vi "Load_TimeTable.vi"(7 "ReadOnly":T11={"Qref"={"ValveCTR"=refnum, "Error"=refnum}, "UI_EN"=FALSE, "UserEventREF"={"TimeBasedProducer"={"Reg"=refnum, "Ref"=refnum}, "TimeBasedTempRead"={"Reg"=refnum, "Ref"=refnum}}, "UI_REF"=variant, "Paths"={"Log_Dir"=path "", "TempLog"=path "", "WateringLog"=path "", "Error"=path "", "Settings_Dir"=path "", "CFG.ini"=path "", "Plant_Digital_OP"=path "", "TimeTable"=path "", "Consol_Dir"=path "", "Input"=path "", "Output"=path "", "Timeout"=path "", "TimeoutTable"=path "", "Ch_Stat"=path "", "Temp"=path ""}, "PI_REF"={"IO"=enum."Remote", "Interface"=enum."Serial", "LINX Device Config"={"Interface"=enum."Serial", "COM Port"="COM13", "TCP Configuration"={"IP Address"="", "Port"=0}, "Device Family"=1, "Device ID"=1, "Device Name"="myRIO-1900", "TCP Ref"=refnum, "Channels"={"DI"=[0, 1, 2, 3, 4, 5, 6, 7, 8, 9, 10, 11, 12, 13, 14, 15, 16, 17, 18, 19, 20, 21, 22, 23, 24, 25, 26, 27, 28, 29, 30, 31, 32, 33, 34, 35, 36, 37, 38, 39, 40, 41, 42, 43, 44, 45, 46], "DO"=[0, 1, 2, 3, 4, 5, 6, 7, 8, 9, 10, 11, 12, 13, 14, 15, 16, 17, 18, 19, 20, 21, 22, 23, 24, 25, 26, 27, 28, 29, 30, 31, 32, 33, 34, 35, 36, 37, 38, 39, 40, 41, 42, 43, 44, 45, 46], "AI"=[0, 1, 2, 3, 4, 5, 6, 7, 8, 9, 10, 11], "AO"=[], "PWM"=[3, 5, 6, 9, 10], "QE"=[], "UART"=[0, 1], "I2C 2"=[0], "SPI"=[0], "CAN"=[], "Servo"=[], "AI Ref (V)"=0.0, "AI Resolution (Bits)"=0, "AO Ref (V)"=0.0, "AO Resolution (Bits)"=0}}}, "CFG"={"ProducerEn_PC"=FALSE, "Producer_PC_ms"=0, "ProducerEn_PI"=FALSE, "Producer_PI_ms"=0, "TempLogInterval"=15, "SystemResetTime"=0.0}} {"CFG"."SystemResetTime" format="%<%H:%M:%S>t"}, 8 "Error In":errorcluster, 10 "Time Table":refnum<vi>, 11 "Read_WriteIN":T1={"Time Table"=[{"Set Time"=0.0, "Control"=enum."Time", "Duration[S]"=3.0, "Liter"=0.0, "Plant Name."="", "Watered"=FALSE, "Su"=FALSE, "Mo"=FALSE, "Tu"=FALSE, "We"=FALSE, "Th"=FALSE, "Fr"=FALSE, "Sa"=FALSE}, {"Set Time"=0.0, "Control"=enum."Time", "Duration[S]"=5.0, "Liter"=0.0, "Plant Name."="", "Watered"=FALSE, "Su"=FALSE, "Mo"=FALSE, "Tu"=FALSE, "We"=FALSE, "Th"=FALSE, "Fr"=FALSE, "Sa"=FALSE}, {"Set Time"=0.0, "Control"=enum."Time", "Duration[S]"=5.0, "Liter"=0.0, "Plant Name."="", "Watered"=FALSE, "Su"=FALSE, "Mo"=FALSE, "Tu"=FALSE, "We"=FALSE, "Th"=FALSE, "Fr"=FALSE, "Sa"=FALSE}], "Plants_Digital_OP"=[], "delta_ms_w_Index"={"delta_ms"=[], "Index"=[], "RunArray"=[]}, "TimeOutInfo"={"Timeout"=0, "ValveCTR"={"State"=enum."Open Valve", "Channel No"=0, "Duration[S]"=0.0}, "Index"=0}, "LoopName"=""} {"TimeOutInfo"."ValveCTR"."Channel No" items=["7"=7, "11"=11, "12"=12, "13"=13, "15"=15, "16"=16, "18"=18, "29"=29, "32"=32, "33"=33, "35"=35, "36"=36, "37"=37, "38"=38, "40"=40]; "delta_ms_w_Index"."RunArray"."Channel No" items=["7"=7, "11"=11, "12"=12, "13"=13, "15"=15, "16"=16, "18"=18, "29"=29, "32"=32, "33"=33, "35"=35, "36"=36, "37"=37, "38"=38, "40"=40]; "Plants_Digital_OP"."Channel No" items=["7"=7, "11"=11, "12"=12, "13"=13, "15"=15, "16"=16, "18"=18, "29"=29, "32"=32, "33"=33, "35"=35, "36"=36, "37"=37, "38"=38, "40"=40]; "Time Table"."Liter" min=0.0; "Time Table"."Set Time" format="%<%H:%M:%S>t"; "Time Table"."Duration[S]" min=0.0}) -> (0 "Error Out":errorcluster, 3 "Read_WriteIOUT":T1={"Time Table"=[{"Set Time"=0.0, "Control"=enum."Time", "Duration[S]"=3.0, "Liter"=0.0, "Plant Name."="", "Watered"=FALSE, "Su"=FALSE, "Mo"=FALSE, "Tu"=FALSE, "We"=FALSE, "Th"=FALSE, "Fr"=FALSE, "Sa"=FALSE}, {"Set Time"=0.0, "Control"=enum."Time", "Duration[S]"=5.0, "Liter"=0.0, "Plant Name."="", "Watered"=FALSE, "Su"=FALSE, "Mo"=FALSE, "Tu"=FALSE, "We"=FALSE, "Th"=FALSE, "Fr"=FALSE, "Sa"=FALSE}, {"Set Time"=0.0, "Control"=enum."Time", "Duration[S]"=5.0, "Liter"=0.0, "Plant Name."="", "Watered"=FALSE, "Su"=FALSE, "Mo"=FALSE, "Tu"=FALSE, "We"=FALSE, "Th"=FALSE, "Fr"=FALSE, "Sa"=FALSE}], "Plants_Digital_OP"=[], "delta_ms_w_Index"={"delta_ms"=[], "Index"=[], "RunArray"=[]}, "TimeOutInfo"={"Timeout"=0, "ValveCTR"={"State"=enum."Open Valve", "Channel No"=0, "Duration[S]"=0.0}, "Index"=0}, "LoopName"=""} {"TimeOutInfo"."ValveCTR"."Channel No" items=["7"=7, "11"=11, "12"=12, "13"=13, "15"=15, "16"=16, "18"=18, "29"=29, "32"=32, "33"=33, "35"=35, "36"=36, "37"=37, "38"=38, "40"=40]; "delta_ms_w_Index"."RunArray"."Channel No" items=["7"=7, "11"=11, "12"=12, "13"=13, "15"=15, "16"=16, "18"=18, "29"=29, "32"=32, "33"=33, "35"=35, "36"=36, "37"=37, "38"=38, "40"=40]; "Plants_Digital_OP"."Channel No" items=["7"=7, "11"=11, "12"=12, "13"=13, "15"=15, "16"=16, "18"=18, "29"=29, "32"=32, "33"=33, "35"=35, "36"=36, "37"=37, "38"=38, "40"=40]; "Time Table"."Liter" min=0.0; "Time Table"."Set Time" format="%<%H:%M:%S>t"; "Time Table"."Duration[S]" min=0.0})   [LabVIEW 2014, in "TimeBasedProd.lvlib"]
uses:
  TimeBasedProd.lvlib
  Main/TypeDef/ReadOnly.ctl
  ValveCTRL/TypeDef/Queue_Cluster.ctl
  ValveCTRL/TypeDef/States_Enum.ctl
  ValveCTRL/TypeDef/CHs_List.ctl
  Main/TypeDef/EventData.ctl
  <vilib>/MakerHub/LINX/Private/Type Defs/LINX Ref.ctl
  <vilib>/MakerHub/LINX/Private/Type Defs/Platform.ctl
  <vilib>/MakerHub/LINX/Private/Type Defs/Interface.ctl
  <vilib>/MakerHub/LINX/Private/Device/Type Defs/LINX Device Config.ctl
  <vilib>/MakerHub/LINX/Private/Device/Type Defs/TCP Config.ctl
  <vilib>/MakerHub/LINX/Private/Device/Type Defs/Channels.ctl
  Main/Init/ReadInitCFG/TypeDef/CFG_Cluster.ctl
  TypeDef/Read_Write.ctl
  TypeDef/Time_Table.ctl
  TypeDef/Time_Table_CTR.ctl
  Digital_OP/TypeDef/Plant_OP_Map.ctl
  Digital_OP/TypeDef/Plant_OP_Map_CTR.ctl
  TypeDef/TimeOutInfo.ctl
  TypeDef/UpdateTimeOutinfo.ctl
  ValveCTRL/ValveCTRL.lvlib
  Main/Main.lvlib
  <vilib>/MakerHub/LINX/LMH-LINX.lvlib
  <vilib>/MakerHub/LINX/Private/Device/Device.lvlib
panel:
  # "Watering Days"
  # "Watering Days"
  # "Watering Days"
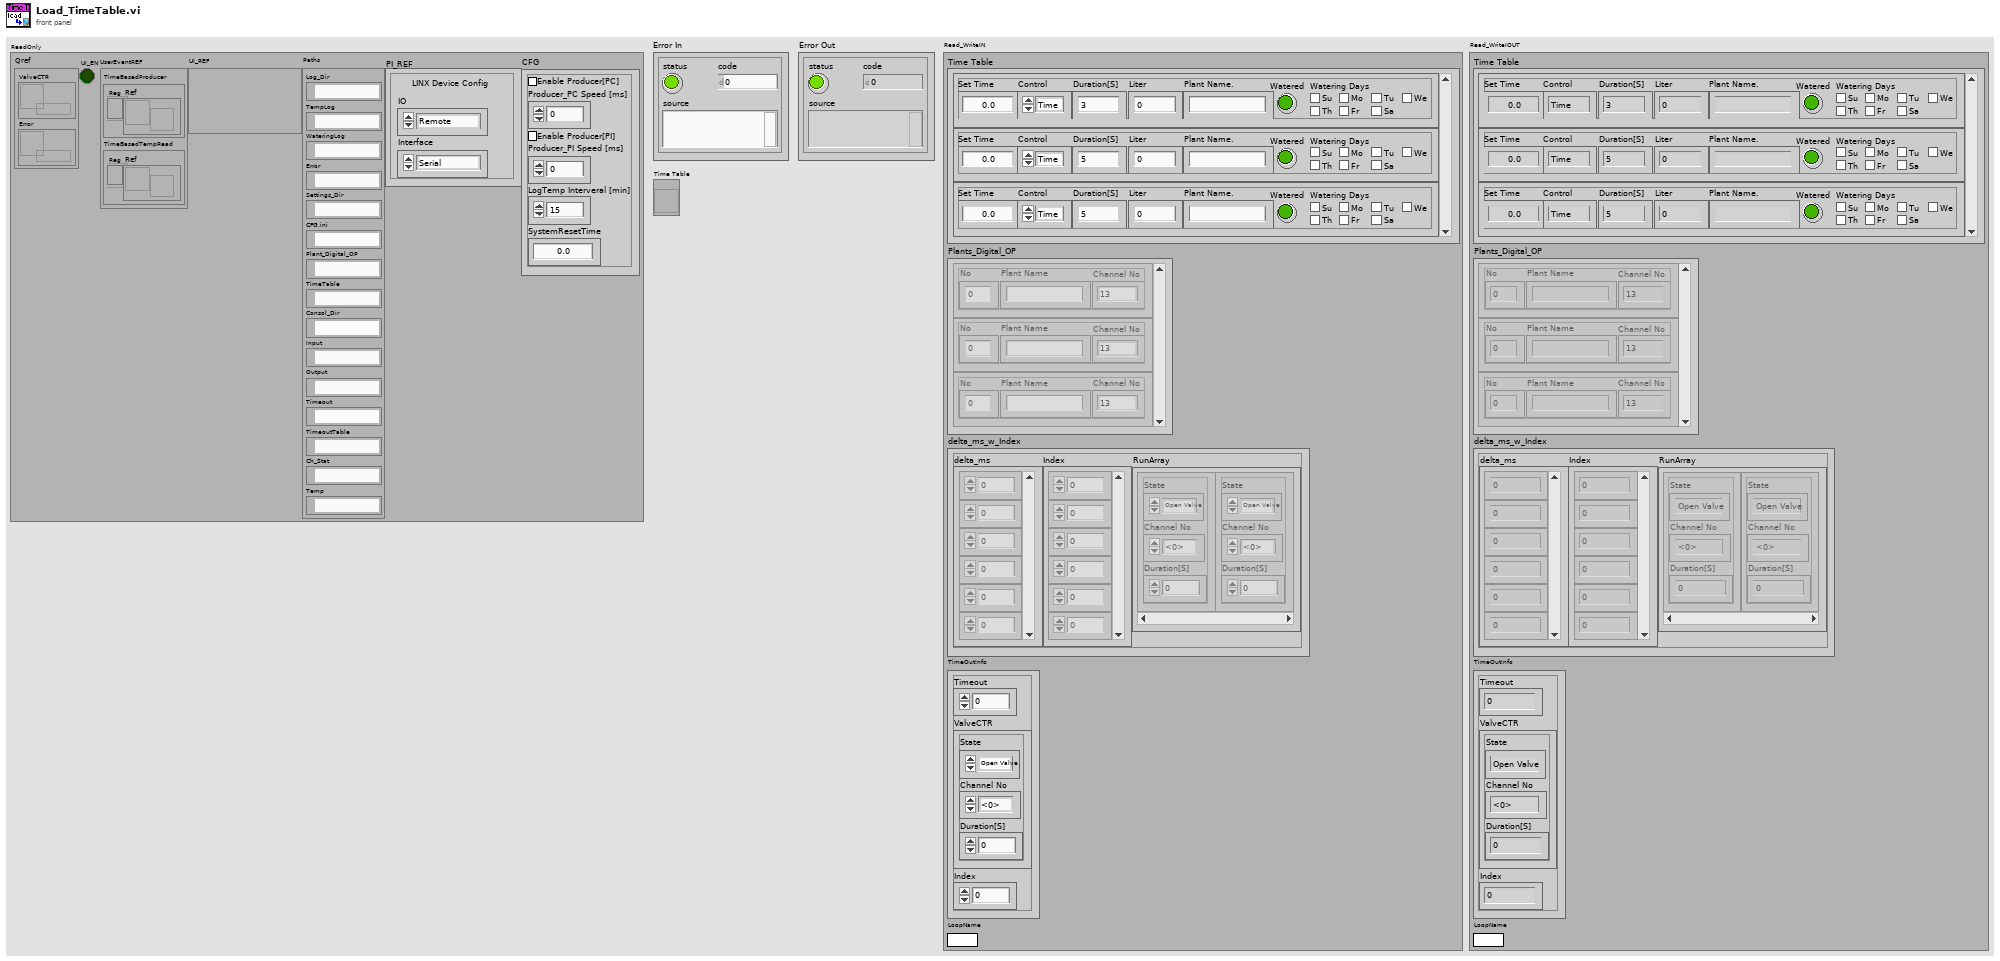
[diagram p1: front panel]
types:
  T1 = typedef "TimeBasedProd.lvlib/Read_Write.ctl" = cluster{"Time Table":T2, "Plants_Digital_OP":T4, "delta_ms_w_Index":T7, "TimeOutInfo":T10, "LoopName":string}
  T2 = typedef "TimeBasedProd.lvlib/Time_Table.ctl" = T3[]
  T3 = typedef "TimeBasedProd.lvlib/Time_Table_CTR.ctl" = cluster{"Set Time":dbl, "Control":enum16{"Time", "Flow"}, "Duration[S]":dbl, "Liter":dbl, "Plant Name.":string, "Watered":bool, "Su":bool, "Mo":bool, "Tu":bool, "We":bool, "Th":bool, "Fr":bool, "Sa":bool}
  T4 = typedef "TimeBasedProd.lvlib/Plant_OP_Map.ctl" = T5[]
  T5 = typedef "TimeBasedProd.lvlib/Plant_OP_Map_CTR.ctl" = cluster{"No":u8, "Plant Name":string, "Channel No":T6}
  T6 = typedef "ValveCTRL.lvlib/CHs_List.ctl" = u8
  T7 = typedef "TimeBasedProd.lvlib/TimeOutInfo.ctl" = cluster{"delta_ms":i32[], "Index":i32[], "RunArray":T8[]}
  T8 = typedef "ValveCTRL.lvlib/Queue_Cluster.ctl" = cluster{"State":T9, "Channel No":T6, "Duration[S]":dbl}
  T9 = typedef "ValveCTRL.lvlib/States_Enum.ctl" = enum16{"Open Pump", "Open Valve", "Wait Valve", "Close Pump", "Close Valve", "Save State", "StopLoop", "ValidCh"}
  T10 = typedef "TimeBasedProd.lvlib/UpdateTimeOutinfo.ctl" = cluster{"Timeout":i32, "ValveCTR":T8, "Index":i32}
  T11 = typedef "Main.lvlib/ReadOnly.ctl" = cluster{"Qref":cluster{"ValveCTR":refnum<queue>, "Error":refnum<queue>}, "UI_EN":bool, "UserEventREF":cluster{"TimeBasedProducer":cluster{"Reg":refnum<event-registration>, "Ref":refnum<user-event>}, "TimeBasedTempRead":cluster{"Reg":refnum<event-registration>, "Ref":refnum<user-event>}}, "UI_REF":variant, "Paths":cluster{"Log_Dir":path, "TempLog":path, "WateringLog":path, "Error":path, "Settings_Dir":path, "CFG.ini":path, "Plant_Digital_OP":path, "TimeTable":path, "Consol_Dir":path, "Input":path, "Output":path, "Timeout":path, "TimeoutTable":path, "Ch_Stat":path, "Temp":path}, "PI_REF":T12, "CFG":T18}
  T12 = typedef "LMH-LINX.lvlib/LINX Ref.ctl" = cluster{"IO":T13, "Interface":T14, "LINX Device Config":T15}
  T13 = typedef "LMH-LINX.lvlib/Platform.ctl" = enum16{"Remote", "Local"}
  T14 = typedef "LMH-LINX.lvlib/Interface.ctl" = enum16{"Serial", "TCP"}
  T15 = typedef "LMH-LINX.lvlib/Device.lvlib/LINX Device Config.ctl" = cluster{"Interface":T14, "COM Port":refnum<visa-resource-name>, "TCP Configuration":T16, "Device Family":u8, "Device ID":u8, "Device Name":string, "TCP Ref":refnum<k5>, "Channels":T17}
  T16 = typedef "LMH-LINX.lvlib/Device.lvlib/TCP Config.ctl" = cluster{"IP Address":string, "Port":u16}
  T17 = typedef "LMH-LINX.lvlib/Channels.ctl" = cluster{"DI":u8[], "DO":u8[], "AI":u8[], "AO":u8[], "PWM":u8[], "QE":u8[], "UART":u8[], "I2C 2":u8[], "SPI":u8[], "CAN":u8[], "Servo":u8[], "AI Ref (V)":dbl, "AI Resolution (Bits)":u8, "AO Ref (V)":dbl, "AO Resolution (Bits)":u8}
  T18 = typedef "Main.lvlib/CFG_Cluster.ctl" = cluster{"ProducerEn_PC":bool, "Producer_PC_ms":u32, "ProducerEn_PI":bool, "Producer_PI_ms":u32, "TempLogInterval":u32, "SystemResetTime":dbl}
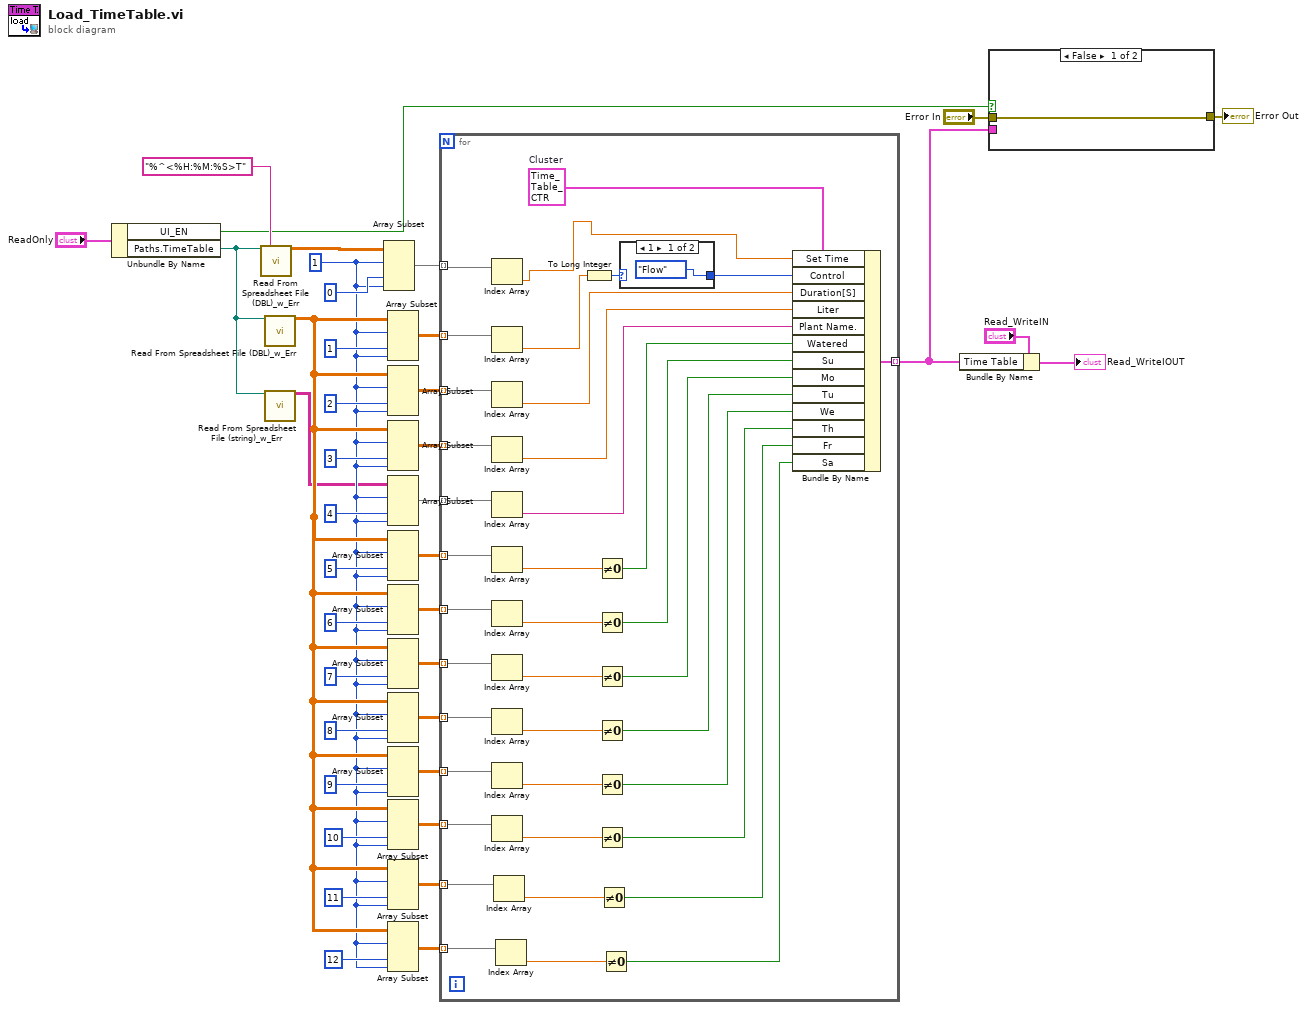
[diagram p0: block diagram]
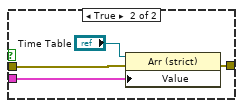
[diagram p2: hidden frame]
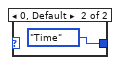
[diagram p3: hidden frame]
diagram:
  w12 = 1 ("index")
  n1 = Unbundle By Name("ReadOnly") -> ("UI_EN"=w2:bool, "Paths.TimeTable"=w8:path)
  n2 = call "Read From Spreadsheet File (DBL)_w_Err.vi"("file path (dialog if empty)"=w8, "format (%.3f)"="%^<%H:%M:%S>T") -> ("all rows"=w36:dbl[][])  [unwired: 8 in, 5 out]
  n3 = call "Read From Spreadsheet File (DBL)_w_Err.vi"("file path (dialog if empty)"=w8) -> ("all rows"=w13:dbl[][])  [unwired: 9 in, 5 out]
  n4 = call "Read From Spreadsheet File (string)_w_Err.vi"("file path (dialog if empty)"=w8) -> ("all rows"=w10:string[][])  [unwired: 9 in, 5 out]
  n5 = Array Subset(array=w36, index (row)=w12, index (col)=0 ("index (row)"), length (col)=w12) -> (w38:dbl[][])  [unwired: 1 in]
  n6 = Array Subset(array=w13, index (row)=w12, index (col)=1 ("index"), length (col)=w12) -> (w35:dbl[][])  [unwired: 1 in]
  n7 = Array Subset(array=w13, index (row)=w12, index (col)=2 ("index"), length (col)=w12) -> (w33:dbl[][])  [unwired: 1 in]
  n8 = Array Subset(array=w13, index (row)=w12, index (col)=3 ("index"), length (col)=w12) -> (w31:dbl[][])  [unwired: 1 in]
  n9 = Array Subset(array=w10, index (row)=w12, index (col)=4 ("index"), length (col)=w12) -> (w29:string[][])  [unwired: 1 in]
  n10 = Array Subset(array=w13, index (row)=w12, index (col)=5 ("index"), length (col)=w12) -> (w27:dbl[][])  [unwired: 1 in]
  n11 = Array Subset(array=w13, index (row)=w12, index (col)=6 ("index"), length (col)=w12) -> (w25:dbl[][])  [unwired: 1 in]
  n12 = Array Subset(array=w13, index (row)=w12, index (col)=7 ("index"), length (col)=w12) -> (w23:dbl[][])  [unwired: 1 in]
  n13 = Array Subset(array=w13, index (row)=w12, index (col)=8 ("index"), length (col)=w12) -> (w19:dbl[][])  [unwired: 1 in]
  n14 = Array Subset(array=w13, index (row)=w12, index (col)=9 ("index"), length (col)=w12) -> (w18:dbl[][])  [unwired: 1 in]
  n15 = Array Subset(array=w13, index (row)=w12, index (col)=10 ("index"), length (col)=w12) -> (w16:dbl[][])  [unwired: 1 in]
  n16 = Array Subset(array=w13, index (row)=w12, index (col)=11 ("index"), length (col)=w12) -> (w14:dbl[][])  [unwired: 1 in]
  n17 = Array Subset(array=w13, index (row)=w12, index (col)=12 ("index"), length (col)=w12) -> (w11:dbl[][])  [unwired: 1 in]
  n18 = for {
    tunnel: w38 -> [w41] mode=indexing
    tunnel: [w77] -> w5 mode=indexing
    tunnel: w35 -> [w76] mode=indexing
    tunnel: w33 -> [w75] mode=indexing
    tunnel: w31 -> [w73] mode=indexing
    tunnel: w29 -> [w71] mode=indexing
    tunnel: w27 -> [w70] mode=indexing
    tunnel: w25 -> [w67] mode=indexing
    tunnel: w23 -> [w63] mode=indexing
    tunnel: w19 -> [w57] mode=indexing
    tunnel: w18 -> [w54] mode=indexing
    tunnel: w16 -> [w51] mode=indexing
    tunnel: w14 -> [w48] mode=indexing
    tunnel: w11 -> [w45] mode=indexing
    w43 = T3 {"Set Time"=0.0, "Control"=enum."Time", "Duration[S]"=3.0, "Liter"=0.0, "Plant Name."="", "Watered"=FALSE, "Su"=FALSE, "Mo"=FALSE, "Tu"=FALSE, "We"=FALSE, "Th"=FALSE, "Fr"=FALSE, "Sa"=FALSE}  # Cluster
    n19 = Index Array(array=w41) -> (element=w40:dbl)  [unwired: 1 in]
    n20 = Index Array(array=w76) -> (element=w59:dbl)  [unwired: 1 in]
    n21 = Index Array(array=w75) -> (element=w74:dbl)  [unwired: 1 in]
    n22 = Index Array(array=w73) -> (element=w72:dbl)  [unwired: 1 in]
    n23 = Index Array(array=w71) -> (element=w42:string)  [unwired: 1 in]
    n24 = Index Array(array=w70) -> (element=w69:dbl)  [unwired: 1 in]
    n25 = Index Array(array=w67) -> (element=w66:dbl)  [unwired: 1 in]
    n26 = Index Array(array=w63) -> (element=w64:dbl)  [unwired: 1 in]
    n27 = Index Array(array=w57) -> (element=w58:dbl)  [unwired: 1 in]
    n28 = Index Array(array=w54) -> (element=w55:dbl)  [unwired: 1 in]
    n29 = Index Array(array=w51) -> (element=w52:dbl)  [unwired: 1 in]
    n30 = Index Array(array=w48) -> (element=w49:dbl)  [unwired: 1 in]
    n31 = Index Array(array=w45) -> (element=w46:dbl)  [unwired: 1 in]
    n32 = To Long Integer(number=w59) -> (32bit integer=w60:i32)
    n33 = Not Equal To 0?(x=w69) -> (x != 0?=w68:bool)
    n34 = Not Equal To 0?(x=w66) -> (x != 0?=w65:bool)
    n35 = Not Equal To 0?(x=w64) -> (x != 0?=w62:bool)
    n36 = Not Equal To 0?(x=w58) -> (x != 0?=w56:bool)
    n37 = Not Equal To 0?(x=w55) -> (x != 0?=w53:bool)
    n38 = Not Equal To 0?(x=w52) -> (x != 0?=w50:bool)
    n39 = Not Equal To 0?(x=w49) -> (x != 0?=w47:bool)
    n40 = Not Equal To 0?(x=w46) -> (x != 0?=w44:bool)
    n41 = case shown="1" w60 {
      tunnel: [enum16{"Time", "Flow"}."Flow" ("Control") enum16{"Time", "Flow"}."Time" ("Control")] -> w61
      frame 1 {
      }
      frame 0, Default {
      }
    }
    n42 = Bundle By Name(cluster=w43, "Set Time"=w40, "Control"=w61, "Duration[S]"=w74, "Liter"=w72, "Plant Name."=w42, "Watered"=w68, "Su"=w65, "Mo"=w62, "Tu"=w56, "We"=w53, "Th"=w50, "Fr"=w47, "Sa"=w44) -> (w77:T3)
  }
  n43 = Bundle By Name(cluster="Read_WriteIN", "Time Table"=w5) -> (→"Read_WriteIOUT":T1)
  n44 = case shown="False" w2 {
    tunnel: w5 -> [_ w84]
    tunnel: [w80 w83] -> w4
    tunnel: "Error In" -> [w80 w81]
    frame False {
    }
    frame True {
      n45 = property class="Arr (strict)"(reference="Time Table", error in=w81, "Value"=w84) -> (error out=w83:errorcluster)  [unwired: 1 out]
    }
  }
  "Error Out" <- w4
